vi "FindDevices.vi"() -> (0 "Devices":T1[](array[typedef]))   [LabVIEW 2010]
uses:
  Controls/SpiDevice.ctl
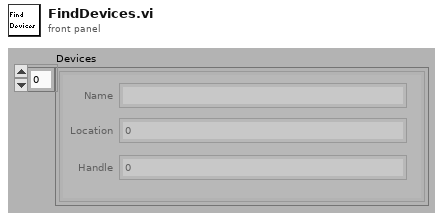
[diagram p1: front panel]
types:
  T1 = typedef "SpiDevice.ctl" = cluster{"Name":string, "Location":u32, "Handle":u32}
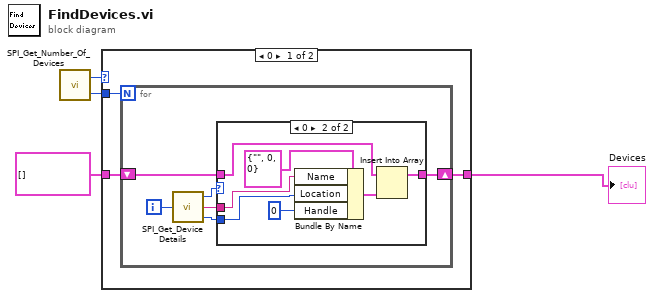
[diagram p0: block diagram]
diagram:
  n1 = call "SPI_Get_Number_Of_Devices.vi"() -> ("NumDevices"=w2:u32, "FTC_Status"=w3:u32)
  n2 = case shown="0" w3 {
    tunnel: w2 -> [w7 _]
    tunnel: T1[] [] -> [w6 w22]
    tunnel: [w5 w22] -> w1
    frame 0 {
      n3 = for {
        N: w7 -> [_]
        shift-right: [w9] -> w5
        shift-left: w6 -> [w10]
        i -> [w13]
        n4 = call "SPI_Get_Device Details.vi"("DeviceIndex"=w13) -> ("FTC_Status"=w8:u32, "DeviceName"=w11:string, "LocID"=w12:u32)
        n5 = case shown="0" w8 {
          tunnel: w12 -> [_ w16]
          tunnel: w11 -> [_ w17]
          tunnel: w10 -> [w14 w21]
          tunnel: [w14 w20] -> w9
          frame Default {
          }
          frame 0 {
            n6 = Bundle By Name(cluster=T1 {"Name"="", "Location"=0, "Handle"=0} ("Device"), "Name"=w17, "Location"=w16, "Handle"=u32 0) -> (w15:T1)
            n7 = Insert Into Array(array=w21, new element=w15) -> (w20:T1[])  [unwired: 1 in]
          }
        }
      }
    }
    frame Default {
    }
  }
  "Devices" <- w1
